vi "LIFA Serial Read Write.vi"() -> ()   [LabVIEW 2023]
uses:
  <vilib>/LabVIEW Interface for Arduino/LabVIEW Interface for Arduino.lvlib
  <vilib>/LabVIEW Interface for Arduino/Type Defs/Board Type.ctl
  <vilib>/LabVIEW Interface for Arduino/Type Defs/Connection Type.ctl
panel:
  out "Read Buffer":string
  out "error out":errorcluster
  in  "error in":errorcluster
  in  "Connection Type (USB/Serial)":T1
  in  "Bytes Per Packet (15)":u32=15
  in  "Board Type (Uno)":T2
  in  "Baud Rate (115200)":u32=115200
  in  "VISA resource":refnum<visa-resource-name>
  in  "stop":bool
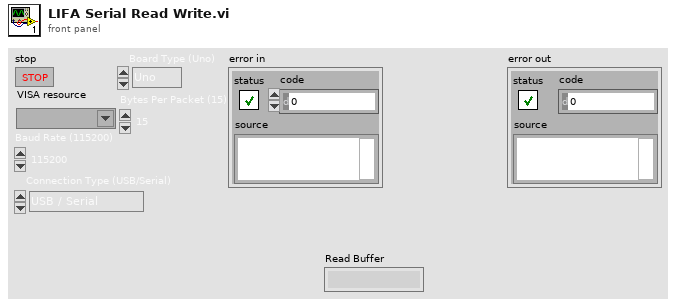
[diagram p1: front panel]
types:
  T1 = typedef "LabVIEW Interface for Arduino.lvlib/Connection Type.ctl" = enum8{"USB / Serial", "XBEE", "BlueSmirf (Bluetooth)"}
  T2 = typedef "LabVIEW Interface for Arduino.lvlib/Board Type.ctl" = enum16{"Uno", "Dimuelanove w/Atmega 328", "Mega 2560"}
  T3 = typedef "LabVIEW Interface for Arduino.lvlib/Arduino Resource.ctl" = cluster{"VISA resource":refnum<visa-resource-name>, "Board Type":T2, "Connection Type":enum8{"USB / Serial"}, "Bytes Per Packet (15)":u8}
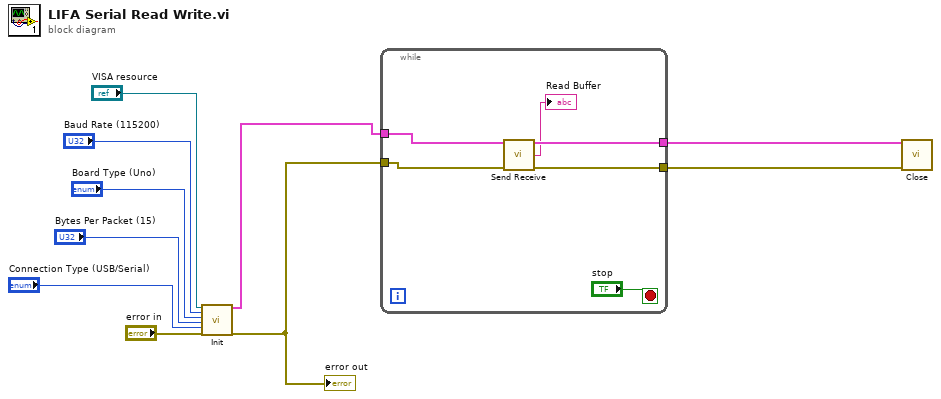
[diagram p0: block diagram]
diagram:
  n1 = call <vilib>:"Init.vi"("VISA resource"="VISA resource", "Baud Rate (115200)"="Baud Rate (115200)", "Board Type (Uno)"="Board Type (Uno)", "Bytes Per Packet (15)"="Bytes Per Packet (15)", "Connection Type (USB/Serial)"="Connection Type (USB/Serial)", "error in"="error in") -> ("Arduino Resource"=w1:T3, "error out"=w2:errorcluster)  [unwired: 12 in]
  "error out" <- w2
  n2 = while {
    tunnel: [w15] -> w4
    tunnel: [w14] -> w3
    tunnel: w2 -> [w12]
    tunnel: w1 -> [w11]
    stop <- "stop" stop-if-true
    n3 = call <vilib>:"Send Receive.vi"("Arduino Resource"=w11, "error in"=w12) -> ("Arduino Resource"=w15:T3, "Read Buffer"=→"Read Buffer":string, "error out"=w14:errorcluster)  [unwired: 11 in]
  }
  n4 = call <vilib>:"Close.vi"("Arduino Resource"=w4, "error in"=w3) -> ()  [unwired: 13 in, 1 out]
